vi "Set Syringe Valve Interlock Configuration.vi"(8 "error in (no error)":errorcluster, 9 "Manual Mode (False)":bool, 10 "Open? (False)":bool, 11 "Syringe Line in":refnum<class "Syringe Line.lvclass">) -> (0 "error out":errorcluster, 1 "Interlock Chain":refnum<class "Interlock Chain.lvclass">, 2 "Open? (False)":bool, 3 "Syringe Line out":refnum<class "Syringe Line.lvclass">)   [LabVIEW 2015, in "cRIO-Carbondioxide.lvlib" / "CO2-Actor.lvlib" / "Syringe Line.lvclass"]
uses:
  Syringe Line.lvclass
  Interlocks/Interlock Chain/Interlock Chain.lvclass
  Interlocks/Interlock/Interlock.lvclass
  Controls/Sample Push State Enumerator.ctl
  Interlocks/Controls/Add IL to -Enumerator.ctl
  Transfer Line/Transfer Line.lvclass
  Interlocks/Interlock Sample/Interlock Sample.lvclass
  subs/Sample/Sample.lvclass
  CO2 Actor Messages/Ping Msg/Ping Msg.lvclass/Ping Msg.ctl
  <vilib>/ActorFramework/Message Enqueuer/Message Enqueuer.lvclass/Message Enqueuer.ctl
  Transfer Line/Transfer Line.lvclass/Transfer Line.ctl
  Interlocks/Interlock Chain/Interlock Chain.lvclass/Interlock Chain.ctl
  <vilib>/ActorFramework/Message Enqueuer/Enqueue.vi
  <vilib>/ActorFramework/Message Priority Queue/Priority Enqueue.vi
  subs/Sample/Read Sample From Container.vi
  CO2 Actor Messages/Ping Msg/Ping Msg.lvclass
  <vilib>/ActorFramework/Actor/Actor.lvclass
  CO2 Actor/CO2 Actor.lvclass
  cRIO-CO2/cRIO-CO2.lvclass
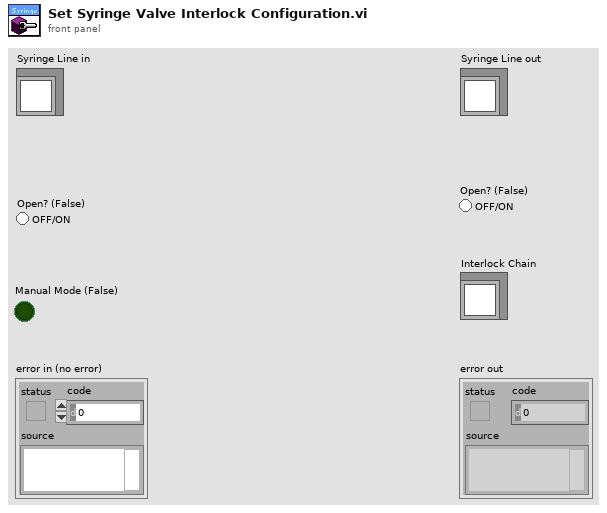
[diagram p1: front panel]
types:
  T1 = typedef "Add IL to -Enumerator.ctl" = enum16{"Deny", "Allow", "None"}
  T2 = typedef "Sample Push State Enumerator.ctl" = enum16{"Undefined", "Initialize", "Dilute", "Close Transfer Line", "Start Heaters", "Warm Up Syringe", "Ready to Push", "Push", "Initiate Stash", "Stash", "Complete", "Abort", "Idle", "Error"}
  T3 = typedef "Dedicated Enqueuers.ctl" = cluster{"Freezers":cluster{"Syringe":refnum<class "Message Enqueuer.lvclass">, "Tank 1":refnum<class "Message Enqueuer.lvclass">, "Tank 2":refnum<class "Message Enqueuer.lvclass">, "Tank 3":refnum<class "Message Enqueuer.lvclass">, "Tank 4":refnum<class "Message Enqueuer.lvclass">}, "Heaters":cluster{"Syringe":refnum<class "Message Enqueuer.lvclass">, "Piston":refnum<class "Message Enqueuer.lvclass">}, "Blowers":cluster{"Tank 1":refnum<class "Message Enqueuer.lvclass">, "Tank 2":refnum<class "Message Enqueuer.lvclass">, "Tank 3":refnum<class "Message Enqueuer.lvclass">, "Tank 4":refnum<class "Message Enqueuer.lvclass">, "Syringe":refnum<class "Message Enqueuer.lvclass">}, "Sample Line":refnum<class "Message Enqueuer.lvclass">, "Storage Line":refnum<class "Message Enqueuer.lvclass">, "Transfer Line":refnum<class "Message Enqueuer.lvclass">, "Syringe Stepper":refnum<class "Message Enqueuer.lvclass">, "Syringe Line":refnum<class "Message Enqueuer.lvclass">, "Capillary Line":refnum<class "Message Enqueuer.lvclass">, "Preparation Line":refnum<class "Message Enqueuer.lvclass">, "Turbo":refnum<class "Message Enqueuer.lvclass">, "Vacuum":refnum<class "Message Enqueuer.lvclass">, "He Line":refnum<class "Message Enqueuer.lvclass">, "Cylinder":refnum<class "Message Enqueuer.lvclass">}
  T4 = typedef "Sample Container.ctl" = cluster{"Sample In":refnum<k21>, "Sample Name":refnum<k21>, "Ti Cathode":refnum<k21>, "SampleQ":refnum<queue>}
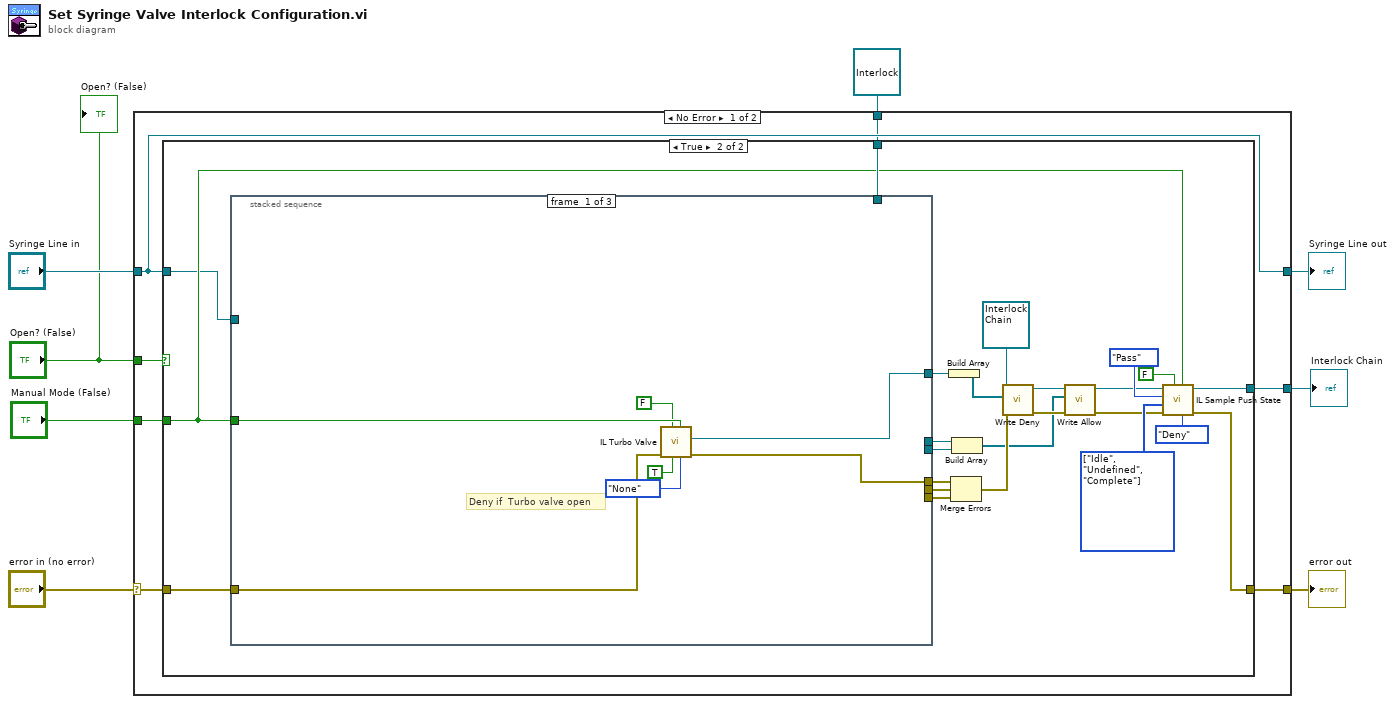
[diagram p0: block diagram]
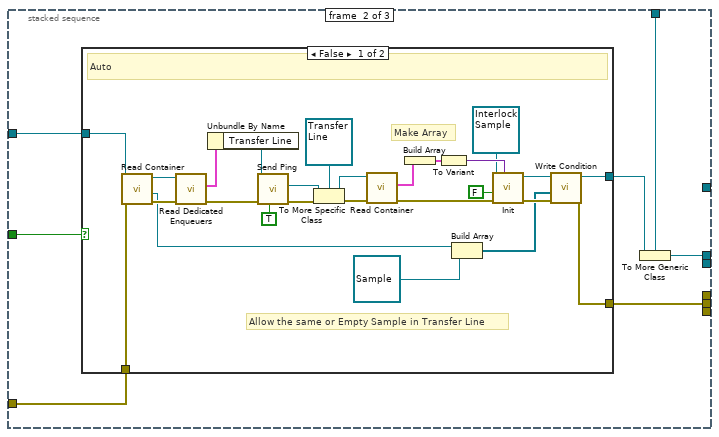
[diagram p3: hidden frame]
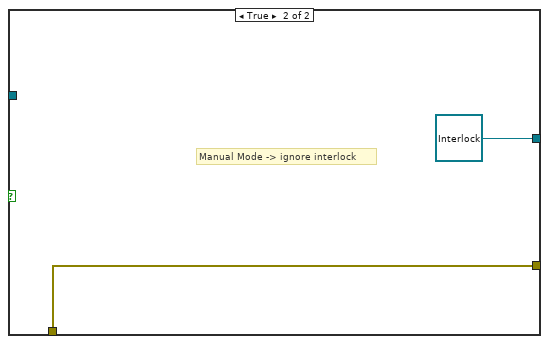
[diagram p4: hidden frame]
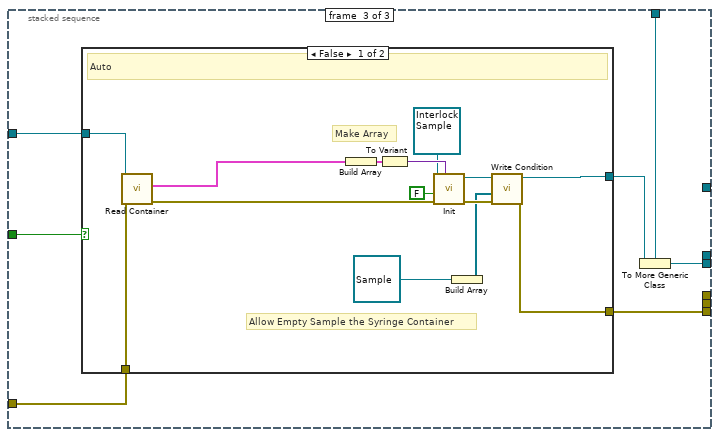
[diagram p5: hidden frame]
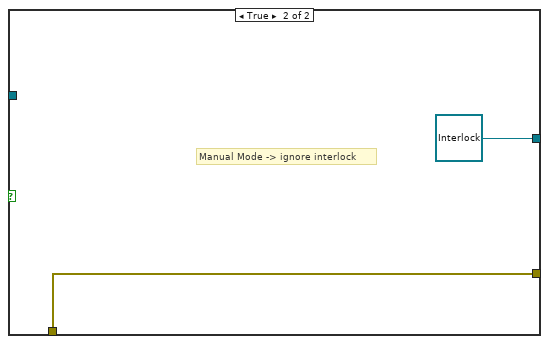
[diagram p6: hidden frame]
diagram:
  n1 = case shown="No Error" "error in (no error)" {
    selector: "error in (no error)" -> [w14 w107]
    tunnel: [w12 w107] -> w7
    tunnel: [w11 w106] -> w5
    tunnel: "Syringe Line in" -> [w11 w106]
    tunnel: "Manual Mode (False)" -> [w15 _]
    tunnel: [w13 _] -> w3
    tunnel: refnum<class "Interlock.lvclass"> refnum ("Interlock.lvclass") -> [w10 _]
    tunnel: "Open? (False)" -> [w9 _]
    frame No Error {
      n2 = case shown="True" w9 {
        tunnel: w15 -> [_ w19]
        tunnel: w14 -> [w16 w40]
        tunnel: [_ w22] -> w13
        tunnel: [w16 w20] -> w12
        tunnel: w11 -> [_ w18]
        tunnel: w10 -> [_ w32]
        frame False {
          # "Close Valve, no interlock"
        }
        frame True {
          w25 = T2[] [enum."Idle", enum."Undefined", enum."Complete"] items=["Undefined", "Initialize", "Dilute", "Close Transfer Line", "Start Heaters", "Warm Up Syringe", "Ready to Push", "Push", "Initiate Stash", "Stash", "Complete", "Abort", "Idle", "Error"] ("States")
          n3 = stacked-sequence {
            tunnel: w19 -> [w43 w54 w89]
            tunnel: w18 -> [_ w53 w88]
            tunnel: w40 -> [w47 w52 w87]
            tunnel: [w45 _ _] -> w37
            tunnel: [w46 _ _] -> w35
            tunnel: w32 -> [_ w50 w85]
            tunnel: [_ w49 _] -> w30
            tunnel: [_ w48 _] -> w31
            tunnel: [_ _ w84] -> w28
            tunnel: [_ _ w83] -> w27
            frame #0 {
              # "Deny if  Turbo valve open"
              n4 = call "IL Turbo Valve.vi"("Add to (Deny)"=Add_IL_to_-Enumerator."None", "Ignore (F)"=w43, "Interlock Condition (ON/OFF)"=TRUE ("Interlock Condition"), "Stop Self on IL? (T)"=FALSE, "error in (no error)"=w47) -> ("error out"=w46:errorcluster, "IL Turbo Valve"=w45:refnum<class "Interlock.lvclass">)  [unwired: 4 in, 1 out]
            }
            frame #1 {
              n5 = case shown="False" w54 {
                tunnel: [w57 w82] -> w48
                tunnel: w53 -> [w75 _]
                tunnel: w52 -> [w73 w82]
                tunnel: [w56 refnum<class "Interlock.lvclass"> refnum ("Interlock.lvclass")] -> w51
                frame False {
                  # "Allow the same or Empty Sample in Transfer Line"
                  # "Make Array"
                  # "Auto"
                  n6 = call "Read Container.vi"("error in (no error)"=w73, "Syringe Line in"=w75) -> ("error out"=w71:errorcluster, "Sample"=w59:refnum<class "Sample.lvclass">, "Syringe Line out"=w74:refnum<class "Syringe Line.lvclass">)  [unwired: 6 in, 1 out]
                  n7 = call "Read Dedicated Enqueuers.vi"("error in (no error)"=w71, "CO2 Actor in"=w74) -> ("error out"=w70:errorcluster, "Dedicated Enqueuers"=w80:T3)  [unwired: 6 in, 2 out]
                  n8 = Unbundle By Name(w80) -> ("Transfer Line"=w79:refnum<class "Message Enqueuer.lvclass">)
                  n9 = call "Send Ping.vi"("Return Self (F)"=TRUE, "error in (no error)"=w70, "Message Enqueuer"=w79) -> ("error out"=w77:errorcluster, "Actor out"=w76:refnum<class "Actor.lvclass">)  [unwired: 5 in, 2 out]
                  n10 = To More Specific Class(target class=refnum<class "Transfer Line.lvclass"> refnum ("Transfer Line.lvclass"), reference=w76, error in=w77) -> (specific class reference=w68:refnum<class "Transfer Line.lvclass">, error out=w69:errorcluster)
                  n11 = call "Read Container.vi"("error in (no error)"=w69, "Transfer Line in"=w68) -> ("error out"=w63:errorcluster, "Sample Container"=w66:T4)  [unwired: 5 in, 3 out]
                  n12 = Build Array(w66) -> (w67:T4[])
                  n13 = To Variant(anything=w67) -> (Variant=w62:variant)
                  n14 = Build Array(w59, refnum<class "Sample.lvclass"> refnum ("Sample.lvclass")) -> (w58:refnum<class "Sample.lvclass">[])
                  n15 = call-dynamic "Init.vi"("Sample Containers SHV (Array!)"=w62, "error in (no error)"=w63, "Stop Self on IL? (T)"=FALSE, "Interlock Sample in"=refnum<class "Interlock Sample.lvclass"> refnum ("Interlock Sample.lvclass")) -> ("error out"=w64:errorcluster, "Interlock Sample out"=w65:refnum<class "Interlock Sample.lvclass">)  [unwired: 6 in]
                  n16 = call "Write Condition.vi"("error in (no error)"=w64, "Samples"=w58, "Interlock Sample in"=w65) -> ("error out"=w57:errorcluster, "Interlock Sample out"=w56:refnum<class "Interlock Sample.lvclass">)  [unwired: 7 in]
                }
                frame True {
                  # "Manual Mode -> ignore interlock"
                }
              }
              n17 = To More Generic Class(target class=w50, reference=w51) -> (generic class reference=w49:refnum<class "Interlock.lvclass">)
            }
            frame #2 {
              n18 = case shown="False" w89 {
                tunnel: [w94 w105] -> w83
                tunnel: w88 -> [w103 _]
                tunnel: w87 -> [w102 w105]
                tunnel: [w93 refnum<class "Interlock.lvclass"> refnum ("Interlock.lvclass")] -> w86
                frame False {
                  # "Allow Empty Sample the Syringe Container"
                  # "Make Array"
                  # "Auto"
                  n19 = call "Read Container.vi"("error in (no error)"=w102, "Syringe Line in"=w103) -> ("error out"=w92:errorcluster, "Container"=w91:T4)  [unwired: 6 in, 2 out]
                  n20 = Build Array(w91) -> (w101:T4[])
                  n21 = To Variant(anything=w101) -> (Variant=w98:variant)
                  n22 = call-dynamic "Init.vi"("Sample Containers SHV (Array!)"=w98, "error in (no error)"=w92, "Stop Self on IL? (T)"=FALSE, "Interlock Sample in"=refnum<class "Interlock Sample.lvclass"> refnum ("Interlock Sample.lvclass")) -> ("error out"=w99:errorcluster, "Interlock Sample out"=w100:refnum<class "Interlock Sample.lvclass">)  [unwired: 6 in]
                  n23 = Build Array(refnum<class "Sample.lvclass"> refnum ("Sample.lvclass")) -> (w95:refnum<class "Sample.lvclass">[])
                  n24 = call "Write Condition.vi"("error in (no error)"=w99, "Samples"=w95, "Interlock Sample in"=w100) -> ("error out"=w94:errorcluster, "Interlock Sample out"=w93:refnum<class "Interlock Sample.lvclass">)  [unwired: 7 in]
                }
                frame True {
                  # "Manual Mode -> ignore interlock"
                }
              }
              n25 = To More Generic Class(target class=w85, reference=w86) -> (generic class reference=w84:refnum<class "Interlock.lvclass">)
            }
          }
          n26 = Build Array(w37) -> (w36:refnum<class "Interlock.lvclass">[])
          n27 = Merge Errors(w35, w31, w27) -> (w34:errorcluster)
          n28 = Build Array(w30, w28) -> (w29:refnum<class "Interlock.lvclass">[])
          n29 = call "Write Deny.vi"("error in (no error)"=w34, "Deny"=w36, "Interlock Chain in"=refnum<class "Interlock Chain.lvclass"> refnum) -> ("error out"=w33:errorcluster, "Interlock Chain out"=w39:refnum<class "Interlock Chain.lvclass">)  [unwired: 7 in]
          n30 = call "Write Allow.vi"("error in (no error)"=w33, "Allow"=w29, "Interlock Chain in"=w39) -> ("error out"=w21:errorcluster, "Interlock Chain out"=w23:refnum<class "Interlock Chain.lvclass">)  [unwired: 7 in]
          n31 = call "IL Sample Push State.vi"("Add to (Deny)"=Add_IL_to_-Enumerator."Deny", "Ignore (F)"=w19, "Stop Self on IL? (T)"=FALSE, "error in (no error)"=w21, "States"=w25, "Pass/Seize"=enum16{"Pass", "Seize"}."Pass", "Interlock Chain in"=w23) -> ("error out"=w20:errorcluster, "Interlock Chain out"=w22:refnum<class "Interlock Chain.lvclass">)  [unwired: 2 in, 1 out]
        }
      }
    }
    frame Error {
    }
  }
  "error out" <- w7
  "Syringe Line out" <- w5
  "Interlock Chain" <- w3
  "Open? (False)" <- "Open? (False)"
